vi "Location Front Panel Defaults.vi"(0 "Debug Mode?":bool, 1 "output cluster":T1, 2 "Location":T2=enum."WCM Main") -> ()   [LabVIEW 2022 SP3]
uses:
  -ScanSystem/Controls/location.ctl
  Motion Controllers/NI_controller/-NI_MotionRoutines/MotionSys.ctl
  -ScanSystem/Controls/Breath_Mode.ctl
  -ScanSystem/Controls/EKG_Mode.ctl
  Digitizers/-DigitizerRoutines/DigConfig.ctl
  Pulsers/pulser.ctl
  Digitizers/-DigitizerRoutines/Digitizer.ctl
  Switch Modules/SwitchOption.ctl
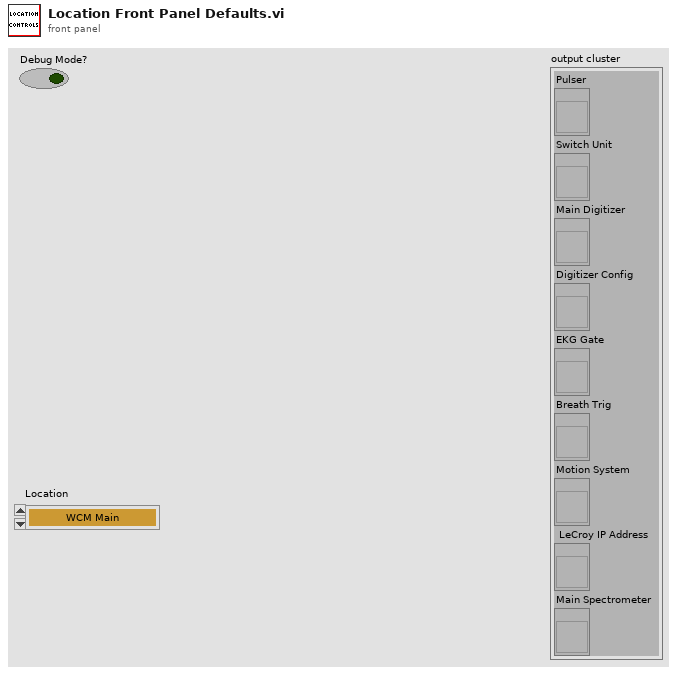
[diagram p1: front panel]
types:
  T1 = cluster{"Pulser":refnum<vi>, "Switch Unit":refnum<vi>, "Main Digitizer":refnum<vi>, "Digitizer Config":refnum<vi>, "EKG Gate":refnum<vi>, "Breath Trig":refnum<vi>, "Motion System":refnum<vi>, " LeCroy IP Address":refnum<vi>, "Main Spectrometer":refnum<vi>}
  T2 = typedef "location.ctl" = enum16{"Automatic", "WCM Main", "Hawaii", "Columbia MM3000", "Columbia  NI System", "NYU", "RRI 2", "UHI Allen", "CUMC RT", "Chiba", "Stony Brook", "WCM Microscopy", "WCM Aeoretch", "WCM Optics Lab", "WCM Main 2Axis", "WCM Rotation", "WCM SAM SMAC", "SERI GP", "SERI SAM 2023"}
  T3 = enum8{"Enabled", "Disabled", "Disabled and Grayed Out"}
  T4 = typedef "Digitizer.ctl" = enum16{"Acqiris Digitizer", "NI Digitizer", "LeCroy", "GaGe", "AlazarTech", "No Digitizer", "Teledyne"}
  T5 = typedef "pulser.ctl" = enum16{"Pan 5900", "Daxsonics", "Agilent 33xxx", "UTEX", "JSR", "WMC Mono-Cycle", "No Pulser", "NYU AVTECH", "Tabor W1281A", "Pan 5800", "Unlisted", "Tabor WX2182B"}
  T6 = typedef "DigConfig.ctl" = enum16{"Single channel", "2 Chans w/ 2 Acqiris", "2 Chans w/ 1 Acqiris", "5-CH Pulser New", "5-CH pulser w/ ann array", "5-pass style ann array", "Empty"}
  T7 = enum16{"Cytex", "Pickering", "NI Switch", "No Switch", "Riverside USB"}
  T8 = typedef "MotionSys.ctl" = enum16{"MM3000", "NI 735x", "Newport ESP", "No Motion Card", "Galil"}
  T9 = typedef "SwitchOption.ctl" = enum16{"Cytex", "Pickering", "NI Switch", "No Switch", "Riverside USB"}
  T10 = typedef "EKG_Mode.ctl" = u16
  T11 = typedef "Breath_Mode.ctl" = u16
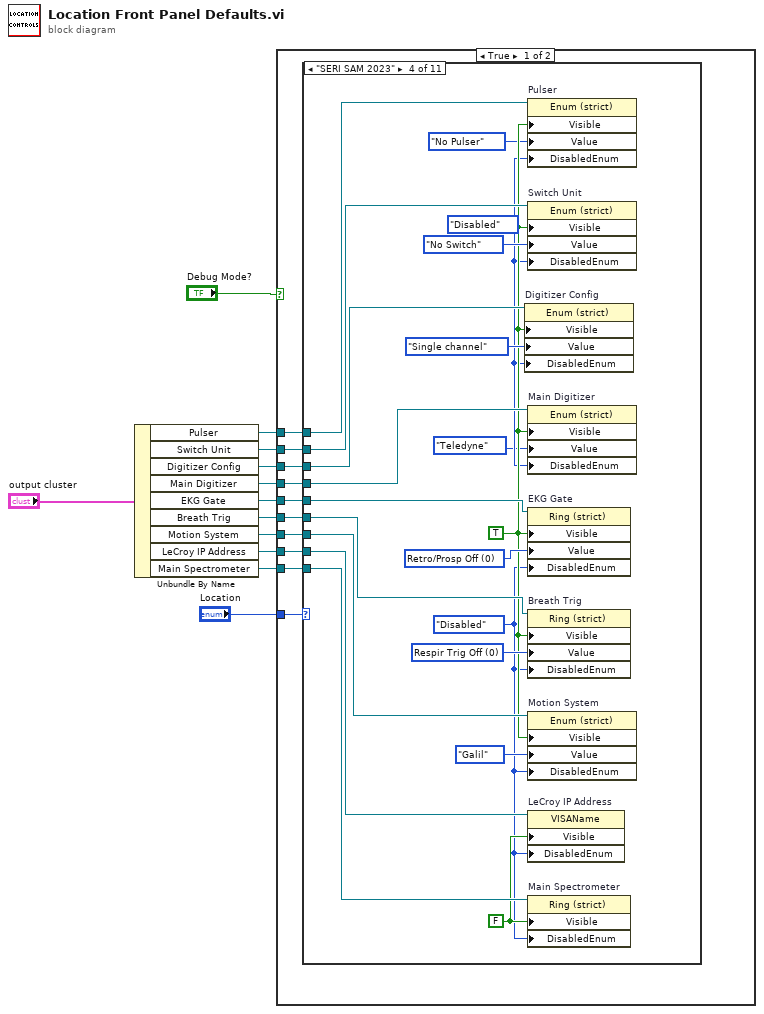
[diagram p0: block diagram]
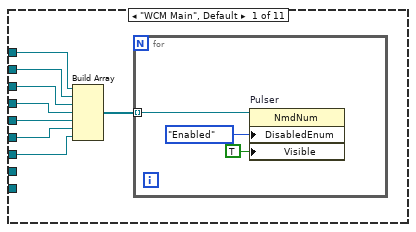
[diagram p2: hidden frame]
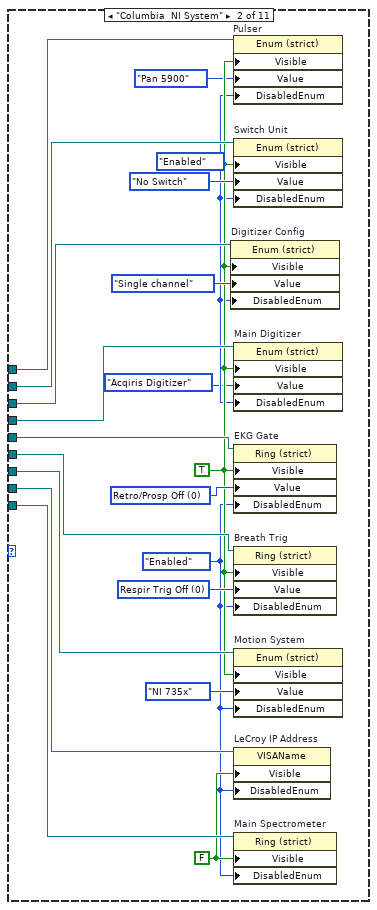
[diagram p3: hidden frame]
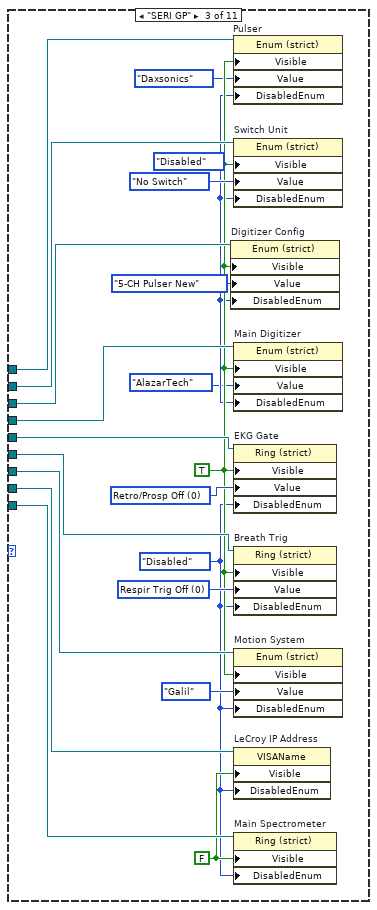
[diagram p4: hidden frame]
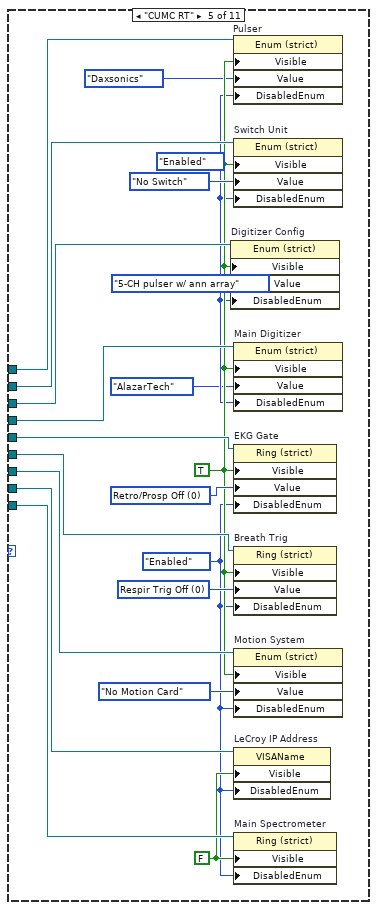
[diagram p5: hidden frame]
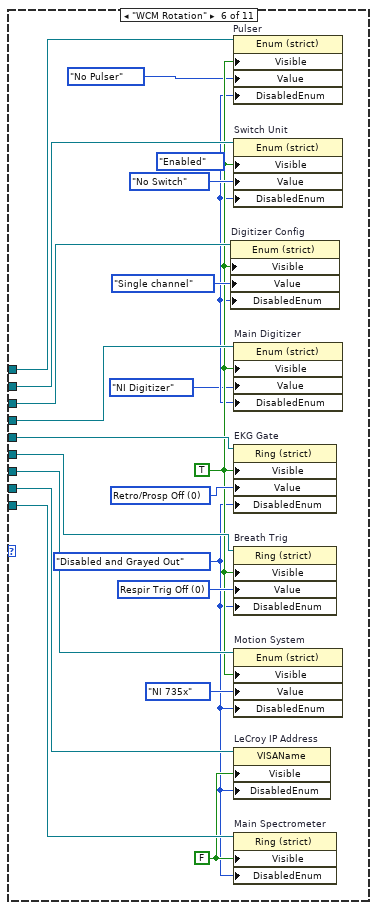
[diagram p6: hidden frame]
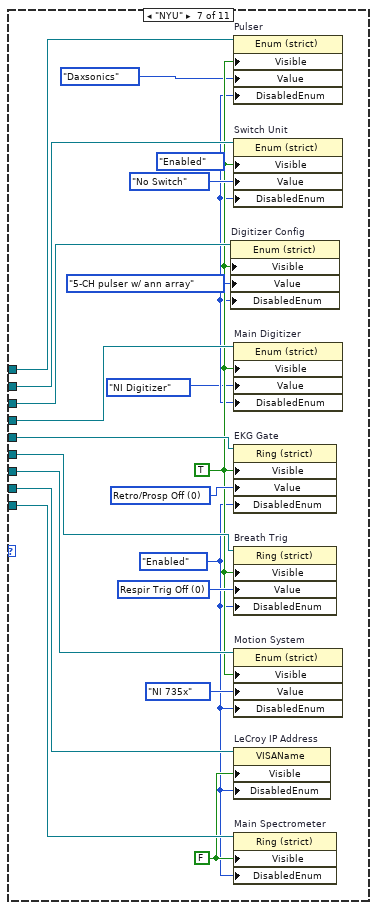
[diagram p7: hidden frame]
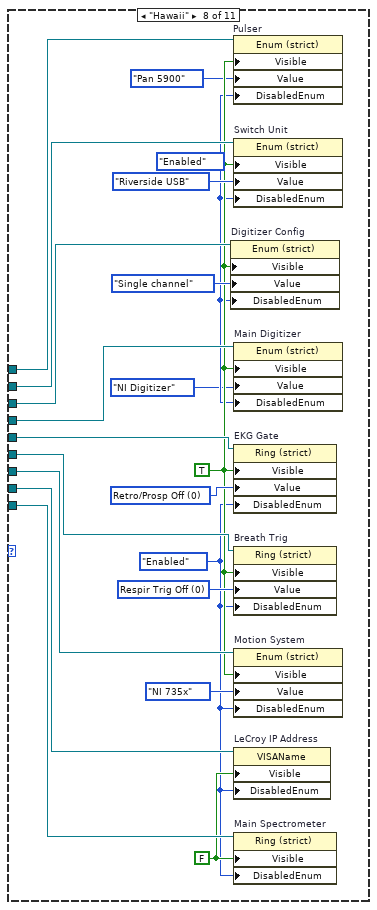
[diagram p8: hidden frame]
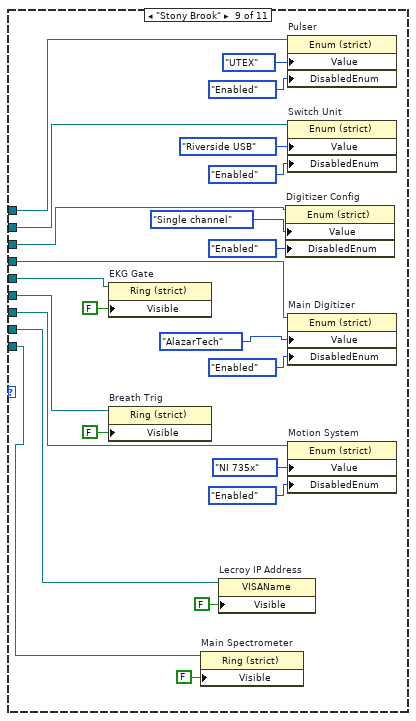
[diagram p9: hidden frame]
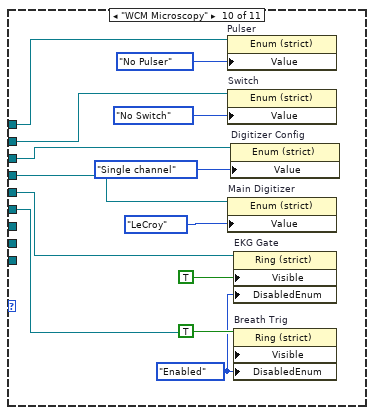
[diagram p10: hidden frame]
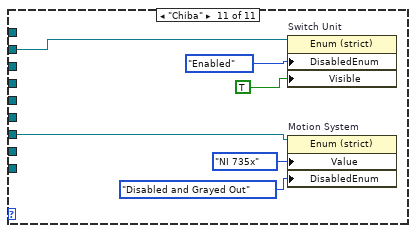
[diagram p11: hidden frame]
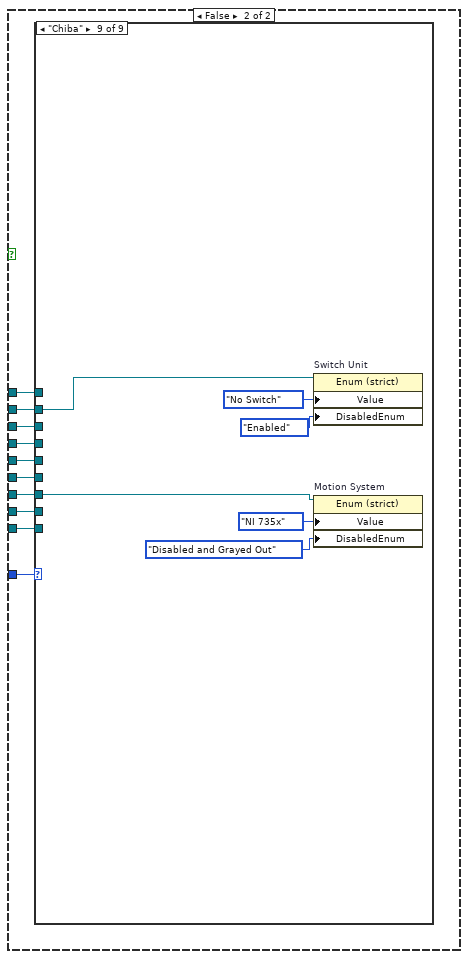
[diagram p12: hidden frame]
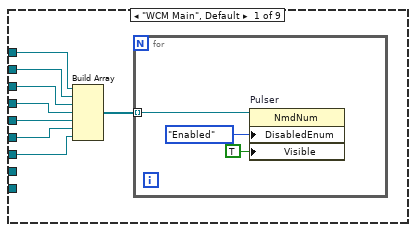
[diagram p13: hidden frame]
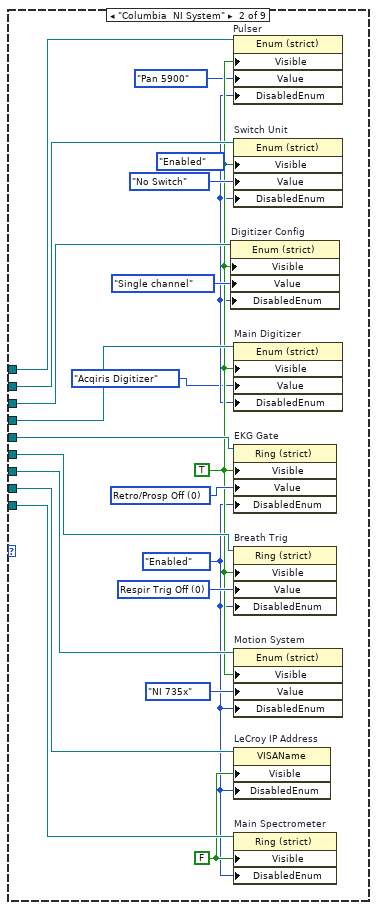
[diagram p14: hidden frame]
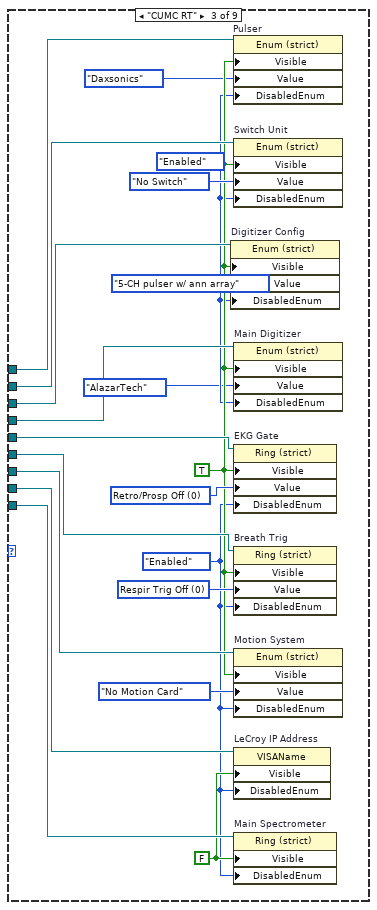
[diagram p15: hidden frame]
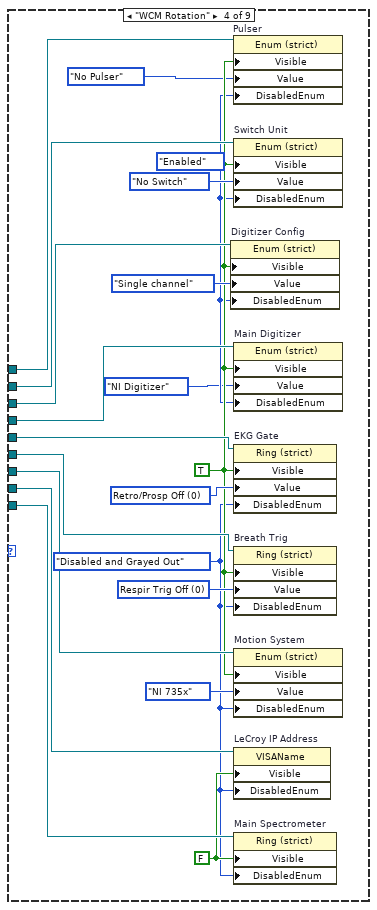
[diagram p16: hidden frame]
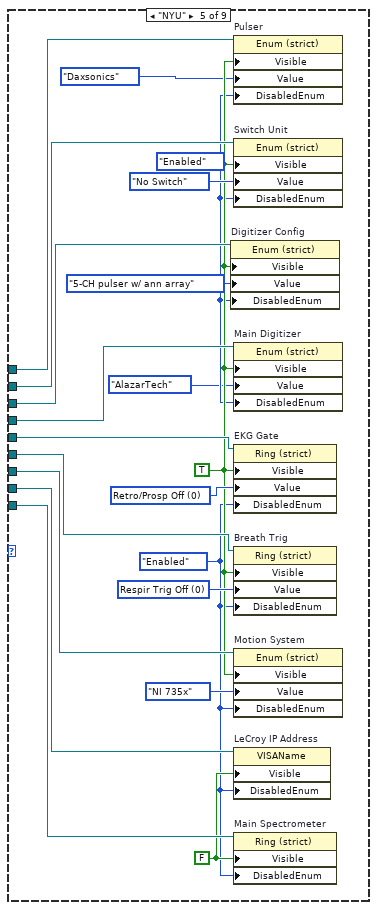
[diagram p17: hidden frame]
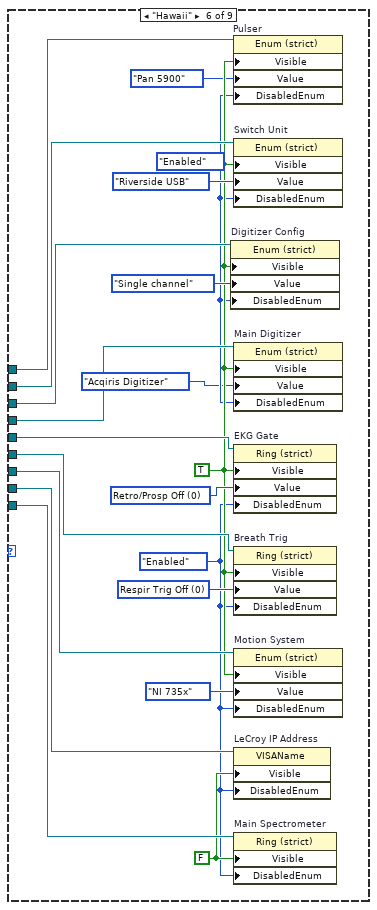
[diagram p18: hidden frame]
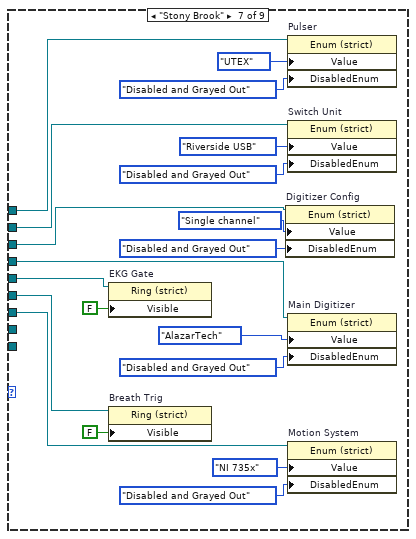
[diagram p19: hidden frame]
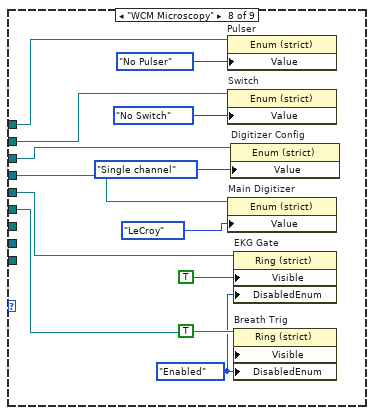
[diagram p20: hidden frame]
diagram:
  n1 = Unbundle By Name("output cluster") -> ("Pulser"=w3:refnum<vi>, "Switch Unit"=w12:refnum<vi>, "Digitizer Config"=w11:refnum<vi>, "Main Digitizer"=w10:refnum<vi>, "EKG Gate"=w9:refnum<vi>, "Breath Trig"=w8:refnum<vi>, "Motion System"=w7:refnum<vi>, "LeCroy IP Address"=w6:refnum<vi>, "Main Spectrometer"=w5:refnum<vi>)
  n2 = case shown="True" "Debug Mode?" {
    tunnel: w12 -> [w22 w225]
    tunnel: w11 -> [w21 w224]
    tunnel: w10 -> [w20 w223]
    tunnel: w9 -> [w19 w222]
    tunnel: w8 -> [w18 w221]
    tunnel: w7 -> [w17 w220]
    tunnel: w6 -> [w16 w219]
    tunnel: w5 -> [w15 w218]
    tunnel: "Location" -> [w14 w217]
    tunnel: w3 -> [w13 w216]
    frame True {
      n3 = case shown="\"SERI SAM 2023\"" w14 {
        tunnel: w13 -> [w30 w53 w73 w93 w113 w133 w153 w173 w195 w209 _]
        tunnel: w22 -> [w29 w52 w72 w92 w112 w132 w152 w172 w192 w200 w214]
        tunnel: w21 -> [w28 w50 w70 w90 w110 w130 w150 w170 w191 w207 _]
        tunnel: w20 -> [w27 w48 w68 w88 w108 w128 w148 w168 w187 w206 _]
        tunnel: w19 -> [w26 w47 w67 w87 w107 w127 w147 w167 w184 w203 _]
        tunnel: w18 -> [w25 w45 w65 w85 w105 w125 w145 w165 w183 w202 _]
        tunnel: w17 -> [w24 w43 w63 w83 w103 w123 w143 w163 w180 _ w213]
        tunnel: w16 -> [_ w40 w60 w80 w100 w120 w140 w160 w178 _ _]
        tunnel: w15 -> [_ w39 w59 w79 w99 w119 w139 w159 w176 _ _]
        frame "WCM Main", Default {
          n4 = Build Array(w30, w29, w28, w27, w26, w25, w24) -> (w23:refnum<vi>[])
          n5 = for {
            tunnel: w23 -> [w32] mode=indexing
            n6 = property on="Pulser" class="NmdNum"(reference=w32, "DisabledEnum"=T3."Enabled" ("Disabled"), "Visible"=TRUE) -> ()  [unwired: 1 in, 2 out]
          }
        }
        frame "Columbia  NI System" {
          w36 = T3."Enabled" ("Disabled")
          w46 = T10 0 items=["Retro/Prosp Off", "Prosp Ext EKG", "Prosp IQ EKG", "Retro EKG", "Retro IQ", "Retro No EKG"] ("Value")
          w44 = T11 0 items=["Respir Trig Off", "Respir Ring1 (Ch1)", "Respir Ch0", "Dig Edge"] ("Value")
          w37 = T3."Enabled" ("Disabled")
          w38 = FALSE
          w41 = TRUE
          n7 = property on="Digitizer Config" class="Enum (strict)"(reference=w50, "Visible"=w41, "Value"=DigConfig."Single channel" ("Dig Config"), "DisabledEnum"=w36) -> ()  [unwired: 1 in, 2 out]
          n8 = property on="Pulser" class="Enum (strict)"(reference=w53, "Visible"=w41, "Value"=pulser."Pan 5900" ("Pulser"), "DisabledEnum"=w36) -> ()  [unwired: 1 in, 2 out]
          n9 = property on="Switch Unit" class="Enum (strict)"(reference=w52, "Visible"=w41, "Value"=T7."No Switch", "DisabledEnum"=w36) -> ()  [unwired: 1 in, 2 out]
          n10 = property on="Main Digitizer" class="Enum (strict)"(reference=w48, "Visible"=w41, "Value"=Digitizer."Acqiris Digitizer", "DisabledEnum"=w36) -> ()  [unwired: 1 in, 2 out]
          n11 = property on="EKG Gate" class="Ring (strict)"(reference=w47, "Visible"=w41, "Value"=w46, "DisabledEnum"=w37) -> ()  [unwired: 1 in, 2 out]
          n12 = property on="Breath Trig" class="Ring (strict)"(reference=w45, "Visible"=w41, "Value"=w44, "DisabledEnum"=w37) -> ()  [unwired: 1 in, 2 out]
          n13 = property on="Motion System" class="Enum (strict)"(reference=w43, "Visible"=w41, "Value"=MotionSys."NI 735x", "DisabledEnum"=w37) -> ()  [unwired: 1 in, 2 out]
          n14 = property on="LeCroy IP Address" class="VISAName"(reference=w40, "Visible"=w38, "DisabledEnum"=w37) -> ()  [unwired: 1 in, 2 out]
          n15 = property on="Main Spectrometer" class="Ring (strict)"(reference=w39, "Visible"=w38, "DisabledEnum"=w37) -> ()  [unwired: 1 in, 2 out]
        }
        frame "SERI GP" {
          w56 = T3."Disabled" ("Disabled")
          w66 = T10 0 items=["Retro/Prosp Off", "Prosp Ext EKG", "Prosp IQ EKG", "Retro EKG", "Retro IQ", "Retro No EKG"] ("Value")
          w64 = T11 0 items=["Respir Trig Off", "Respir Ring1 (Ch1)", "Respir Ch0", "Dig Edge"] ("Value")
          w57 = T3."Disabled" ("Disabled")
          w58 = FALSE
          w61 = TRUE
          n16 = property on="Digitizer Config" class="Enum (strict)"(reference=w70, "Visible"=w61, "Value"=DigConfig."5-CH Pulser New" ("Dig Config"), "DisabledEnum"=w56) -> ()  [unwired: 1 in, 2 out]
          n17 = property on="Pulser" class="Enum (strict)"(reference=w73, "Visible"=w61, "Value"=pulser."Daxsonics" ("Pulser"), "DisabledEnum"=w56) -> ()  [unwired: 1 in, 2 out]
          n18 = property on="Switch Unit" class="Enum (strict)"(reference=w72, "Visible"=w61, "Value"=T7."No Switch", "DisabledEnum"=w56) -> ()  [unwired: 1 in, 2 out]
          n19 = property on="Main Digitizer" class="Enum (strict)"(reference=w68, "Visible"=w61, "Value"=Digitizer."AlazarTech", "DisabledEnum"=w56) -> ()  [unwired: 1 in, 2 out]
          n20 = property on="EKG Gate" class="Ring (strict)"(reference=w67, "Visible"=w61, "Value"=w66, "DisabledEnum"=w57) -> ()  [unwired: 1 in, 2 out]
          n21 = property on="Breath Trig" class="Ring (strict)"(reference=w65, "Visible"=w61, "Value"=w64, "DisabledEnum"=w57) -> ()  [unwired: 1 in, 2 out]
          n22 = property on="Motion System" class="Enum (strict)"(reference=w63, "Visible"=w61, "Value"=MotionSys."Galil", "DisabledEnum"=w57) -> ()  [unwired: 1 in, 2 out]
          n23 = property on="LeCroy IP Address" class="VISAName"(reference=w60, "Visible"=w58, "DisabledEnum"=w57) -> ()  [unwired: 1 in, 2 out]
          n24 = property on="Main Spectrometer" class="Ring (strict)"(reference=w59, "Visible"=w58, "DisabledEnum"=w57) -> ()  [unwired: 1 in, 2 out]
        }
        frame "SERI SAM 2023" {
          w76 = T3."Disabled" ("Disabled")
          w86 = T10 0 items=["Retro/Prosp Off", "Prosp Ext EKG", "Prosp IQ EKG", "Retro EKG", "Retro IQ", "Retro No EKG"] ("Value")
          w84 = T11 0 items=["Respir Trig Off", "Respir Ring1 (Ch1)", "Respir Ch0", "Dig Edge"] ("Value")
          w77 = T3."Disabled" ("Disabled")
          w78 = FALSE
          w81 = TRUE
          n25 = property on="Digitizer Config" class="Enum (strict)"(reference=w90, "Visible"=w81, "Value"=DigConfig."Single channel" ("Dig Config"), "DisabledEnum"=w76) -> ()  [unwired: 1 in, 2 out]
          n26 = property on="Pulser" class="Enum (strict)"(reference=w93, "Visible"=w81, "Value"=pulser."No Pulser" ("Pulser"), "DisabledEnum"=w76) -> ()  [unwired: 1 in, 2 out]
          n27 = property on="Switch Unit" class="Enum (strict)"(reference=w92, "Visible"=w81, "Value"=T7."No Switch", "DisabledEnum"=w76) -> ()  [unwired: 1 in, 2 out]
          n28 = property on="Main Digitizer" class="Enum (strict)"(reference=w88, "Visible"=w81, "Value"=Digitizer."Teledyne", "DisabledEnum"=w76) -> ()  [unwired: 1 in, 2 out]
          n29 = property on="EKG Gate" class="Ring (strict)"(reference=w87, "Visible"=w81, "Value"=w86, "DisabledEnum"=w77) -> ()  [unwired: 1 in, 2 out]
          n30 = property on="Breath Trig" class="Ring (strict)"(reference=w85, "Visible"=w81, "Value"=w84, "DisabledEnum"=w77) -> ()  [unwired: 1 in, 2 out]
          n31 = property on="Motion System" class="Enum (strict)"(reference=w83, "Visible"=w81, "Value"=MotionSys."Galil", "DisabledEnum"=w77) -> ()  [unwired: 1 in, 2 out]
          n32 = property on="LeCroy IP Address" class="VISAName"(reference=w80, "Visible"=w78, "DisabledEnum"=w77) -> ()  [unwired: 1 in, 2 out]
          n33 = property on="Main Spectrometer" class="Ring (strict)"(reference=w79, "Visible"=w78, "DisabledEnum"=w77) -> ()  [unwired: 1 in, 2 out]
        }
        frame "CUMC RT" {
          w96 = T3."Enabled" ("Disabled")
          w106 = T10 0 items=["Retro/Prosp Off", "Prosp Ext EKG", "Prosp IQ EKG", "Retro EKG", "Retro IQ", "Retro No EKG"] ("Value")
          w104 = T11 0 items=["Respir Trig Off", "Respir Ring1 (Ch1)", "Respir Ch0", "Dig Edge"] ("Value")
          w97 = T3."Enabled" ("Disabled")
          w98 = FALSE
          w101 = TRUE
          n34 = property on="Digitizer Config" class="Enum (strict)"(reference=w110, "Visible"=w101, "Value"=DigConfig."5-CH pulser w/ ann array" ("Dig Config"), "DisabledEnum"=w96) -> ()  [unwired: 1 in, 2 out]
          n35 = property on="Pulser" class="Enum (strict)"(reference=w113, "Visible"=w101, "Value"=pulser."Daxsonics" ("Pulser"), "DisabledEnum"=w96) -> ()  [unwired: 1 in, 2 out]
          n36 = property on="Switch Unit" class="Enum (strict)"(reference=w112, "Visible"=w101, "Value"=T7."No Switch", "DisabledEnum"=w96) -> ()  [unwired: 1 in, 2 out]
          n37 = property on="Main Digitizer" class="Enum (strict)"(reference=w108, "Visible"=w101, "Value"=Digitizer."AlazarTech", "DisabledEnum"=w96) -> ()  [unwired: 1 in, 2 out]
          n38 = property on="EKG Gate" class="Ring (strict)"(reference=w107, "Visible"=w101, "Value"=w106, "DisabledEnum"=w97) -> ()  [unwired: 1 in, 2 out]
          n39 = property on="Breath Trig" class="Ring (strict)"(reference=w105, "Visible"=w101, "Value"=w104, "DisabledEnum"=w97) -> ()  [unwired: 1 in, 2 out]
          n40 = property on="Motion System" class="Enum (strict)"(reference=w103, "Visible"=w101, "Value"=MotionSys."No Motion Card", "DisabledEnum"=w97) -> ()  [unwired: 1 in, 2 out]
          n41 = property on="LeCroy IP Address" class="VISAName"(reference=w100, "Visible"=w98, "DisabledEnum"=w97) -> ()  [unwired: 1 in, 2 out]
          n42 = property on="Main Spectrometer" class="Ring (strict)"(reference=w99, "Visible"=w98, "DisabledEnum"=w97) -> ()  [unwired: 1 in, 2 out]
        }
        frame "WCM Rotation" {
          w116 = T3."Enabled" ("Disabled")
          w126 = T10 0 items=["Retro/Prosp Off", "Prosp Ext EKG", "Prosp IQ EKG", "Retro EKG", "Retro IQ", "Retro No EKG"] ("Value")
          w124 = T11 0 items=["Respir Trig Off", "Respir Ring1 (Ch1)", "Respir Ch0", "Dig Edge"] ("Value")
          w117 = T3."Disabled and Grayed Out" ("Disabled")
          w118 = FALSE
          w121 = TRUE
          n43 = property on="Digitizer Config" class="Enum (strict)"(reference=w130, "Visible"=w121, "Value"=DigConfig."Single channel" ("Dig Config"), "DisabledEnum"=w116) -> ()  [unwired: 1 in, 2 out]
          n44 = property on="Pulser" class="Enum (strict)"(reference=w133, "Visible"=w121, "Value"=pulser."No Pulser" ("Pulser"), "DisabledEnum"=w116) -> ()  [unwired: 1 in, 2 out]
          n45 = property on="Switch Unit" class="Enum (strict)"(reference=w132, "Visible"=w121, "Value"=T7."No Switch", "DisabledEnum"=w116) -> ()  [unwired: 1 in, 2 out]
          n46 = property on="Main Digitizer" class="Enum (strict)"(reference=w128, "Visible"=w121, "Value"=Digitizer."NI Digitizer", "DisabledEnum"=w116) -> ()  [unwired: 1 in, 2 out]
          n47 = property on="EKG Gate" class="Ring (strict)"(reference=w127, "Visible"=w121, "Value"=w126, "DisabledEnum"=w117) -> ()  [unwired: 1 in, 2 out]
          n48 = property on="Breath Trig" class="Ring (strict)"(reference=w125, "Visible"=w121, "Value"=w124, "DisabledEnum"=w117) -> ()  [unwired: 1 in, 2 out]
          n49 = property on="Motion System" class="Enum (strict)"(reference=w123, "Visible"=w121, "Value"=MotionSys."NI 735x", "DisabledEnum"=w117) -> ()  [unwired: 1 in, 2 out]
          n50 = property on="LeCroy IP Address" class="VISAName"(reference=w120, "Visible"=w118, "DisabledEnum"=w117) -> ()  [unwired: 1 in, 2 out]
          n51 = property on="Main Spectrometer" class="Ring (strict)"(reference=w119, "Visible"=w118, "DisabledEnum"=w117) -> ()  [unwired: 1 in, 2 out]
        }
        frame "NYU" {
          w136 = T3."Enabled" ("Disabled")
          w146 = T10 0 items=["Retro/Prosp Off", "Prosp Ext EKG", "Prosp IQ EKG", "Retro EKG", "Retro IQ", "Retro No EKG"] ("Value")
          w144 = T11 0 items=["Respir Trig Off", "Respir Ring1 (Ch1)", "Respir Ch0", "Dig Edge"] ("Value")
          w137 = T3."Enabled" ("Disabled")
          w138 = FALSE
          w141 = TRUE
          n52 = property on="Digitizer Config" class="Enum (strict)"(reference=w150, "Visible"=w141, "Value"=DigConfig."5-CH pulser w/ ann array" ("Dig Config"), "DisabledEnum"=w136) -> ()  [unwired: 1 in, 2 out]
          n53 = property on="Pulser" class="Enum (strict)"(reference=w153, "Visible"=w141, "Value"=pulser."Daxsonics" ("Pulser"), "DisabledEnum"=w136) -> ()  [unwired: 1 in, 2 out]
          n54 = property on="Switch Unit" class="Enum (strict)"(reference=w152, "Visible"=w141, "Value"=T7."No Switch", "DisabledEnum"=w136) -> ()  [unwired: 1 in, 2 out]
          n55 = property on="Main Digitizer" class="Enum (strict)"(reference=w148, "Visible"=w141, "Value"=Digitizer."NI Digitizer", "DisabledEnum"=w136) -> ()  [unwired: 1 in, 2 out]
          n56 = property on="EKG Gate" class="Ring (strict)"(reference=w147, "Visible"=w141, "Value"=w146, "DisabledEnum"=w137) -> ()  [unwired: 1 in, 2 out]
          n57 = property on="Breath Trig" class="Ring (strict)"(reference=w145, "Visible"=w141, "Value"=w144, "DisabledEnum"=w137) -> ()  [unwired: 1 in, 2 out]
          n58 = property on="Motion System" class="Enum (strict)"(reference=w143, "Visible"=w141, "Value"=MotionSys."NI 735x", "DisabledEnum"=w137) -> ()  [unwired: 1 in, 2 out]
          n59 = property on="LeCroy IP Address" class="VISAName"(reference=w140, "Visible"=w138, "DisabledEnum"=w137) -> ()  [unwired: 1 in, 2 out]
          n60 = property on="Main Spectrometer" class="Ring (strict)"(reference=w139, "Visible"=w138, "DisabledEnum"=w137) -> ()  [unwired: 1 in, 2 out]
        }
        frame "Hawaii" {
          w156 = T3."Enabled" ("Disabled")
          w166 = T10 0 items=["Retro/Prosp Off", "Prosp Ext EKG", "Prosp IQ EKG", "Retro EKG", "Retro IQ", "Retro No EKG"] ("Value")
          w164 = T11 0 items=["Respir Trig Off", "Respir Ring1 (Ch1)", "Respir Ch0", "Dig Edge"] ("Value")
          w157 = T3."Enabled" ("Disabled")
          w158 = FALSE
          w161 = TRUE
          n61 = property on="Digitizer Config" class="Enum (strict)"(reference=w170, "Visible"=w161, "Value"=DigConfig."Single channel" ("Dig Config"), "DisabledEnum"=w156) -> ()  [unwired: 1 in, 2 out]
          n62 = property on="Pulser" class="Enum (strict)"(reference=w173, "Visible"=w161, "Value"=pulser."Pan 5900" ("Pulser"), "DisabledEnum"=w156) -> ()  [unwired: 1 in, 2 out]
          n63 = property on="Switch Unit" class="Enum (strict)"(reference=w172, "Visible"=w161, "Value"=T7."Riverside USB", "DisabledEnum"=w156) -> ()  [unwired: 1 in, 2 out]
          n64 = property on="Main Digitizer" class="Enum (strict)"(reference=w168, "Visible"=w161, "Value"=Digitizer."NI Digitizer", "DisabledEnum"=w156) -> ()  [unwired: 1 in, 2 out]
          n65 = property on="EKG Gate" class="Ring (strict)"(reference=w167, "Visible"=w161, "Value"=w166, "DisabledEnum"=w157) -> ()  [unwired: 1 in, 2 out]
          n66 = property on="Breath Trig" class="Ring (strict)"(reference=w165, "Visible"=w161, "Value"=w164, "DisabledEnum"=w157) -> ()  [unwired: 1 in, 2 out]
          n67 = property on="Motion System" class="Enum (strict)"(reference=w163, "Visible"=w161, "Value"=MotionSys."NI 735x", "DisabledEnum"=w157) -> ()  [unwired: 1 in, 2 out]
          n68 = property on="LeCroy IP Address" class="VISAName"(reference=w160, "Visible"=w158, "DisabledEnum"=w157) -> ()  [unwired: 1 in, 2 out]
          n69 = property on="Main Spectrometer" class="Ring (strict)"(reference=w159, "Visible"=w158, "DisabledEnum"=w157) -> ()  [unwired: 1 in, 2 out]
        }
        frame "Stony Brook" {
          n70 = property on="EKG Gate" class="Ring (strict)"(reference=w184, "Visible"=FALSE) -> ()  [unwired: 1 in, 2 out]
          n71 = property on="Breath Trig" class="Ring (strict)"(reference=w183, "Visible"=FALSE) -> ()  [unwired: 1 in, 2 out]
          n72 = property on="Main Spectrometer" class="Ring (strict)"(reference=w176, "Visible"=FALSE) -> ()  [unwired: 1 in, 2 out]
          n73 = property on="Lecroy IP Address" class="VISAName"(reference=w178, "Visible"=FALSE) -> ()  [unwired: 1 in, 2 out]
          n74 = property on="Digitizer Config" class="Enum (strict)"(reference=w191, "Value"=DigConfig."Single channel" ("Dig Config"), "DisabledEnum"=T3."Enabled" ("Disabled")) -> ()  [unwired: 1 in, 2 out]
          n75 = property on="Pulser" class="Enum (strict)"(reference=w195, "Value"=pulser."UTEX" ("Pulser"), "DisabledEnum"=T3."Enabled" ("Disabled")) -> ()  [unwired: 1 in, 2 out]
          n76 = property on="Switch Unit" class="Enum (strict)"(reference=w192, "Value"=SwitchOption."Riverside USB", "DisabledEnum"=T3."Enabled" ("Disabled")) -> ()  [unwired: 1 in, 2 out]
          n77 = property on="Main Digitizer" class="Enum (strict)"(reference=w187, "Value"=Digitizer."AlazarTech", "DisabledEnum"=T3."Enabled" ("Disabled")) -> ()  [unwired: 1 in, 2 out]
          n78 = property on="Motion System" class="Enum (strict)"(reference=w180, "Value"=MotionSys."NI 735x", "DisabledEnum"=T3."Enabled" ("Disabled")) -> ()  [unwired: 1 in, 2 out]
        }
        frame "WCM Microscopy" {
          w198 = T3."Enabled" ("Disabled")
          n79 = property on="Pulser" class="Enum (strict)"(reference=w209, "Value"=pulser."No Pulser" ("Pulser")) -> ()  [unwired: 1 in, 2 out]
          n80 = property on="Switch" class="Enum (strict)"(reference=w200, "Value"=SwitchOption."No Switch") -> ()  [unwired: 1 in, 2 out]
          n81 = property on="Main Digitizer" class="Enum (strict)"(reference=w206, "Value"=Digitizer."LeCroy") -> ()  [unwired: 1 in, 2 out]
          n82 = property on="Digitizer Config" class="Enum (strict)"(reference=w207, "Value"=DigConfig."Single channel" ("Dig Config")) -> ()  [unwired: 1 in, 2 out]
          n83 = property on="EKG Gate" class="Ring (strict)"(reference=w203, "Visible"=TRUE, "DisabledEnum"=w198) -> ()  [unwired: 1 in, 2 out]
          n84 = property on="Breath Trig" class="Ring (strict)"(reference=w202, "Visible"=TRUE, "DisabledEnum"=w198) -> ()  [unwired: 1 in, 2 out]
        }
        frame "Chiba" {
          n85 = property on="Switch Unit" class="Enum (strict)"(reference=w214, "DisabledEnum"=T3."Enabled" ("Disabled"), "Visible"=TRUE) -> ()  [unwired: 1 in, 2 out]
          n86 = property on="Motion System" class="Enum (strict)"(reference=w213, "Value"=MotionSys."NI 735x", "DisabledEnum"=T3."Disabled and Grayed Out" ("Disabled")) -> ()  [unwired: 1 in, 2 out]
        }
      }
    }
    frame False {
      n87 = case shown="\"Chiba\"" w217 {
        tunnel: w216 -> [w233 w256 w276 w296 w316 w336 w354 w368 _]
        tunnel: w225 -> [w232 w255 w275 w295 w315 w335 w351 w359 w372]
        tunnel: w224 -> [w231 w253 w273 w293 w313 w333 w350 w366 _]
        tunnel: w223 -> [w230 w251 w271 w291 w311 w331 w346 w365 _]
        tunnel: w222 -> [w229 w250 w270 w290 w310 w330 w343 w362 _]
        tunnel: w221 -> [w228 w248 w268 w288 w308 w328 w342 w361 _]
        tunnel: w220 -> [w227 w246 w266 w286 w306 w326 w339 _ w371]
        tunnel: w219 -> [_ w243 w263 w283 w303 w323 _ _ _]
        tunnel: w218 -> [_ w242 w262 w282 w302 w322 _ _ _]
        frame "WCM Main", Default {
          n88 = Build Array(w233, w232, w231, w230, w229, w228, w227) -> (w226:refnum<vi>[])
          n89 = for {
            tunnel: w226 -> [w235] mode=indexing
            n90 = property on="Pulser" class="NmdNum"(reference=w235, "DisabledEnum"=T3."Enabled" ("Disabled"), "Visible"=TRUE) -> ()  [unwired: 1 in, 2 out]
          }
        }
        frame "Columbia  NI System" {
          w239 = T3."Enabled" ("Disabled")
          w249 = T10 0 items=["Retro/Prosp Off", "Prosp Ext EKG", "Prosp IQ EKG", "Retro EKG", "Retro IQ", "Retro No EKG"] ("Value")
          w247 = T11 0 items=["Respir Trig Off", "Respir Ring1 (Ch1)", "Respir Ch0", "Dig Edge"] ("Value")
          w240 = T3."Enabled" ("Disabled")
          w241 = FALSE
          w244 = TRUE
          n91 = property on="Digitizer Config" class="Enum (strict)"(reference=w253, "Visible"=w244, "Value"=DigConfig."Single channel" ("Dig Config"), "DisabledEnum"=w239) -> ()  [unwired: 1 in, 2 out]
          n92 = property on="Pulser" class="Enum (strict)"(reference=w256, "Visible"=w244, "Value"=pulser."Pan 5900" ("Pulser"), "DisabledEnum"=w239) -> ()  [unwired: 1 in, 2 out]
          n93 = property on="Switch Unit" class="Enum (strict)"(reference=w255, "Visible"=w244, "Value"=T7."No Switch", "DisabledEnum"=w239) -> ()  [unwired: 1 in, 2 out]
          n94 = property on="Main Digitizer" class="Enum (strict)"(reference=w251, "Visible"=w244, "Value"=Digitizer."Acqiris Digitizer", "DisabledEnum"=w239) -> ()  [unwired: 1 in, 2 out]
          n95 = property on="EKG Gate" class="Ring (strict)"(reference=w250, "Visible"=w244, "Value"=w249, "DisabledEnum"=w240) -> ()  [unwired: 1 in, 2 out]
          n96 = property on="Breath Trig" class="Ring (strict)"(reference=w248, "Visible"=w244, "Value"=w247, "DisabledEnum"=w240) -> ()  [unwired: 1 in, 2 out]
          n97 = property on="Motion System" class="Enum (strict)"(reference=w246, "Visible"=w244, "Value"=MotionSys."NI 735x", "DisabledEnum"=w240) -> ()  [unwired: 1 in, 2 out]
          n98 = property on="LeCroy IP Address" class="VISAName"(reference=w243, "Visible"=w241, "DisabledEnum"=w240) -> ()  [unwired: 1 in, 2 out]
          n99 = property on="Main Spectrometer" class="Ring (strict)"(reference=w242, "Visible"=w241, "DisabledEnum"=w240) -> ()  [unwired: 1 in, 2 out]
        }
        frame "CUMC RT" {
          w259 = T3."Enabled" ("Disabled")
          w269 = T10 0 items=["Retro/Prosp Off", "Prosp Ext EKG", "Prosp IQ EKG", "Retro EKG", "Retro IQ", "Retro No EKG"] ("Value")
          w267 = T11 0 items=["Respir Trig Off", "Respir Ring1 (Ch1)", "Respir Ch0", "Dig Edge"] ("Value")
          w260 = T3."Enabled" ("Disabled")
          w261 = FALSE
          w264 = TRUE
          n100 = property on="Digitizer Config" class="Enum (strict)"(reference=w273, "Visible"=w264, "Value"=DigConfig."5-CH pulser w/ ann array" ("Dig Config"), "DisabledEnum"=w259) -> ()  [unwired: 1 in, 2 out]
          n101 = property on="Pulser" class="Enum (strict)"(reference=w276, "Visible"=w264, "Value"=pulser."Daxsonics" ("Pulser"), "DisabledEnum"=w259) -> ()  [unwired: 1 in, 2 out]
          n102 = property on="Switch Unit" class="Enum (strict)"(reference=w275, "Visible"=w264, "Value"=T7."No Switch", "DisabledEnum"=w259) -> ()  [unwired: 1 in, 2 out]
          n103 = property on="Main Digitizer" class="Enum (strict)"(reference=w271, "Visible"=w264, "Value"=Digitizer."AlazarTech", "DisabledEnum"=w259) -> ()  [unwired: 1 in, 2 out]
          n104 = property on="EKG Gate" class="Ring (strict)"(reference=w270, "Visible"=w264, "Value"=w269, "DisabledEnum"=w260) -> ()  [unwired: 1 in, 2 out]
          n105 = property on="Breath Trig" class="Ring (strict)"(reference=w268, "Visible"=w264, "Value"=w267, "DisabledEnum"=w260) -> ()  [unwired: 1 in, 2 out]
          n106 = property on="Motion System" class="Enum (strict)"(reference=w266, "Visible"=w264, "Value"=MotionSys."No Motion Card", "DisabledEnum"=w260) -> ()  [unwired: 1 in, 2 out]
          n107 = property on="LeCroy IP Address" class="VISAName"(reference=w263, "Visible"=w261, "DisabledEnum"=w260) -> ()  [unwired: 1 in, 2 out]
          n108 = property on="Main Spectrometer" class="Ring (strict)"(reference=w262, "Visible"=w261, "DisabledEnum"=w260) -> ()  [unwired: 1 in, 2 out]
        }
        frame "WCM Rotation" {
          w279 = T3."Enabled" ("Disabled")
          w289 = T10 0 items=["Retro/Prosp Off", "Prosp Ext EKG", "Prosp IQ EKG", "Retro EKG", "Retro IQ", "Retro No EKG"] ("Value")
          w287 = T11 0 items=["Respir Trig Off", "Respir Ring1 (Ch1)", "Respir Ch0", "Dig Edge"] ("Value")
          w280 = T3."Disabled and Grayed Out" ("Disabled")
          w281 = FALSE
          w284 = TRUE
          n109 = property on="Digitizer Config" class="Enum (strict)"(reference=w293, "Visible"=w284, "Value"=DigConfig."Single channel" ("Dig Config"), "DisabledEnum"=w279) -> ()  [unwired: 1 in, 2 out]
          n110 = property on="Pulser" class="Enum (strict)"(reference=w296, "Visible"=w284, "Value"=pulser."No Pulser" ("Pulser"), "DisabledEnum"=w279) -> ()  [unwired: 1 in, 2 out]
          n111 = property on="Switch Unit" class="Enum (strict)"(reference=w295, "Visible"=w284, "Value"=T7."No Switch", "DisabledEnum"=w279) -> ()  [unwired: 1 in, 2 out]
          n112 = property on="Main Digitizer" class="Enum (strict)"(reference=w291, "Visible"=w284, "Value"=Digitizer."NI Digitizer", "DisabledEnum"=w279) -> ()  [unwired: 1 in, 2 out]
          n113 = property on="EKG Gate" class="Ring (strict)"(reference=w290, "Visible"=w284, "Value"=w289, "DisabledEnum"=w280) -> ()  [unwired: 1 in, 2 out]
          n114 = property on="Breath Trig" class="Ring (strict)"(reference=w288, "Visible"=w284, "Value"=w287, "DisabledEnum"=w280) -> ()  [unwired: 1 in, 2 out]
          n115 = property on="Motion System" class="Enum (strict)"(reference=w286, "Visible"=w284, "Value"=MotionSys."NI 735x", "DisabledEnum"=w280) -> ()  [unwired: 1 in, 2 out]
          n116 = property on="LeCroy IP Address" class="VISAName"(reference=w283, "Visible"=w281, "DisabledEnum"=w280) -> ()  [unwired: 1 in, 2 out]
          n117 = property on="Main Spectrometer" class="Ring (strict)"(reference=w282, "Visible"=w281, "DisabledEnum"=w280) -> ()  [unwired: 1 in, 2 out]
        }
        frame "NYU" {
          w299 = T3."Enabled" ("Disabled")
          w309 = T10 0 items=["Retro/Prosp Off", "Prosp Ext EKG", "Prosp IQ EKG", "Retro EKG", "Retro IQ", "Retro No EKG"] ("Value")
          w307 = T11 0 items=["Respir Trig Off", "Respir Ring1 (Ch1)", "Respir Ch0", "Dig Edge"] ("Value")
          w300 = T3."Enabled" ("Disabled")
          w301 = FALSE
          w304 = TRUE
          n118 = property on="Digitizer Config" class="Enum (strict)"(reference=w313, "Visible"=w304, "Value"=DigConfig."5-CH pulser w/ ann array" ("Dig Config"), "DisabledEnum"=w299) -> ()  [unwired: 1 in, 2 out]
          n119 = property on="Pulser" class="Enum (strict)"(reference=w316, "Visible"=w304, "Value"=pulser."Daxsonics" ("Pulser"), "DisabledEnum"=w299) -> ()  [unwired: 1 in, 2 out]
          n120 = property on="Switch Unit" class="Enum (strict)"(reference=w315, "Visible"=w304, "Value"=T7."No Switch", "DisabledEnum"=w299) -> ()  [unwired: 1 in, 2 out]
          n121 = property on="Main Digitizer" class="Enum (strict)"(reference=w311, "Visible"=w304, "Value"=Digitizer."AlazarTech", "DisabledEnum"=w299) -> ()  [unwired: 1 in, 2 out]
          n122 = property on="EKG Gate" class="Ring (strict)"(reference=w310, "Visible"=w304, "Value"=w309, "DisabledEnum"=w300) -> ()  [unwired: 1 in, 2 out]
          n123 = property on="Breath Trig" class="Ring (strict)"(reference=w308, "Visible"=w304, "Value"=w307, "DisabledEnum"=w300) -> ()  [unwired: 1 in, 2 out]
          n124 = property on="Motion System" class="Enum (strict)"(reference=w306, "Visible"=w304, "Value"=MotionSys."NI 735x", "DisabledEnum"=w300) -> ()  [unwired: 1 in, 2 out]
          n125 = property on="LeCroy IP Address" class="VISAName"(reference=w303, "Visible"=w301, "DisabledEnum"=w300) -> ()  [unwired: 1 in, 2 out]
          n126 = property on="Main Spectrometer" class="Ring (strict)"(reference=w302, "Visible"=w301, "DisabledEnum"=w300) -> ()  [unwired: 1 in, 2 out]
        }
        frame "Hawaii" {
          w319 = T3."Enabled" ("Disabled")
          w329 = T10 0 items=["Retro/Prosp Off", "Prosp Ext EKG", "Prosp IQ EKG", "Retro EKG", "Retro IQ", "Retro No EKG"] ("Value")
          w327 = T11 0 items=["Respir Trig Off", "Respir Ring1 (Ch1)", "Respir Ch0", "Dig Edge"] ("Value")
          w320 = T3."Enabled" ("Disabled")
          w321 = FALSE
          w324 = TRUE
          n127 = property on="Digitizer Config" class="Enum (strict)"(reference=w333, "Visible"=w324, "Value"=DigConfig."Single channel" ("Dig Config"), "DisabledEnum"=w319) -> ()  [unwired: 1 in, 2 out]
          n128 = property on="Pulser" class="Enum (strict)"(reference=w336, "Visible"=w324, "Value"=pulser."Pan 5900" ("Pulser"), "DisabledEnum"=w319) -> ()  [unwired: 1 in, 2 out]
          n129 = property on="Switch Unit" class="Enum (strict)"(reference=w335, "Visible"=w324, "Value"=T7."Riverside USB", "DisabledEnum"=w319) -> ()  [unwired: 1 in, 2 out]
          n130 = property on="Main Digitizer" class="Enum (strict)"(reference=w331, "Visible"=w324, "Value"=Digitizer."Acqiris Digitizer", "DisabledEnum"=w319) -> ()  [unwired: 1 in, 2 out]
          n131 = property on="EKG Gate" class="Ring (strict)"(reference=w330, "Visible"=w324, "Value"=w329, "DisabledEnum"=w320) -> ()  [unwired: 1 in, 2 out]
          n132 = property on="Breath Trig" class="Ring (strict)"(reference=w328, "Visible"=w324, "Value"=w327, "DisabledEnum"=w320) -> ()  [unwired: 1 in, 2 out]
          n133 = property on="Motion System" class="Enum (strict)"(reference=w326, "Visible"=w324, "Value"=MotionSys."NI 735x", "DisabledEnum"=w320) -> ()  [unwired: 1 in, 2 out]
          n134 = property on="LeCroy IP Address" class="VISAName"(reference=w323, "Visible"=w321, "DisabledEnum"=w320) -> ()  [unwired: 1 in, 2 out]
          n135 = property on="Main Spectrometer" class="Ring (strict)"(reference=w322, "Visible"=w321, "DisabledEnum"=w320) -> ()  [unwired: 1 in, 2 out]
        }
        frame "Stony Brook" {
          n136 = property on="EKG Gate" class="Ring (strict)"(reference=w343, "Visible"=FALSE) -> ()  [unwired: 1 in, 2 out]
          n137 = property on="Breath Trig" class="Ring (strict)"(reference=w342, "Visible"=FALSE) -> ()  [unwired: 1 in, 2 out]
          n138 = property on="Digitizer Config" class="Enum (strict)"(reference=w350, "Value"=DigConfig."Single channel" ("Dig Config"), "DisabledEnum"=T3."Disabled and Grayed Out" ("Disabled")) -> ()  [unwired: 1 in, 2 out]
          n139 = property on="Pulser" class="Enum (strict)"(reference=w354, "Value"=pulser."UTEX" ("Pulser"), "DisabledEnum"=T3."Disabled and Grayed Out" ("Disabled")) -> ()  [unwired: 1 in, 2 out]
          n140 = property on="Switch Unit" class="Enum (strict)"(reference=w351, "Value"=SwitchOption."Riverside USB", "DisabledEnum"=T3."Disabled and Grayed Out" ("Disabled")) -> ()  [unwired: 1 in, 2 out]
          n141 = property on="Main Digitizer" class="Enum (strict)"(reference=w346, "Value"=Digitizer."AlazarTech", "DisabledEnum"=T3."Disabled and Grayed Out" ("Disabled")) -> ()  [unwired: 1 in, 2 out]
          n142 = property on="Motion System" class="Enum (strict)"(reference=w339, "Value"=MotionSys."NI 735x", "DisabledEnum"=T3."Disabled and Grayed Out" ("Disabled")) -> ()  [unwired: 1 in, 2 out]
        }
        frame "WCM Microscopy" {
          w357 = T3."Enabled" ("Disabled")
          n143 = property on="Pulser" class="Enum (strict)"(reference=w368, "Value"=pulser."No Pulser" ("Pulser")) -> ()  [unwired: 1 in, 2 out]
          n144 = property on="Switch" class="Enum (strict)"(reference=w359, "Value"=SwitchOption."No Switch") -> ()  [unwired: 1 in, 2 out]
          n145 = property on="Main Digitizer" class="Enum (strict)"(reference=w365, "Value"=Digitizer."LeCroy") -> ()  [unwired: 1 in, 2 out]
          n146 = property on="Digitizer Config" class="Enum (strict)"(reference=w366, "Value"=DigConfig."Single channel" ("Dig Config")) -> ()  [unwired: 1 in, 2 out]
          n147 = property on="EKG Gate" class="Ring (strict)"(reference=w362, "Visible"=TRUE, "DisabledEnum"=w357) -> ()  [unwired: 1 in, 2 out]
          n148 = property on="Breath Trig" class="Ring (strict)"(reference=w361, "Visible"=TRUE, "DisabledEnum"=w357) -> ()  [unwired: 1 in, 2 out]
        }
        frame "Chiba" {
          n149 = property on="Switch Unit" class="Enum (strict)"(reference=w372, "Value"=T7."No Switch", "DisabledEnum"=T3."Enabled" ("Disabled")) -> ()  [unwired: 1 in, 2 out]
          n150 = property on="Motion System" class="Enum (strict)"(reference=w371, "Value"=MotionSys."NI 735x", "DisabledEnum"=T3."Disabled and Grayed Out" ("Disabled")) -> ()  [unwired: 1 in, 2 out]
        }
      }
    }
  }
